vi "Channel Info by Index.vi"(8 "error in (no error)":errorcluster, 10 "Index":i32, 11 "GroupAbstract in":refnum<class "Group.lvclass">) -> (0 "error out":errorcluster, 2 "Channel Info":T1, 3 "GroupAbstract out":refnum<class "Group.lvclass">)   [LabVIEW 2020, in "Vecto.lvlib" / "Group.lvclass"]
uses:
  Group.lvclass
  Channel Info.ctl
  Group.lvclass/Group.ctl
  VectoConfig/VectoConfig.lvlib
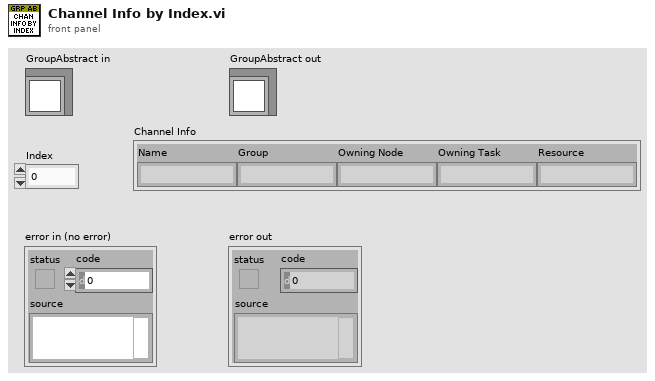
[diagram p1: front panel]
types:
  T1 = typedef "VectoConfig.lvlib/Channel Info.ctl" = cluster{"Name":string, "Group":string, "Owning Node":string, "Owning Task":string, "Resource":string}
  T2 = typedef "Vecto.lvlib/GroupAbstract.lvclass/Ref.ctl" = cluster{"Channel Index Map":map{string, i32}, "Channel Info":T3[]}
  T3 = typedef "Vecto.lvlib/Channel Info.ctl" = cluster{"Name":string, "Group":string, "Owning Node":string, "Owning Task":string, "Resource":string}
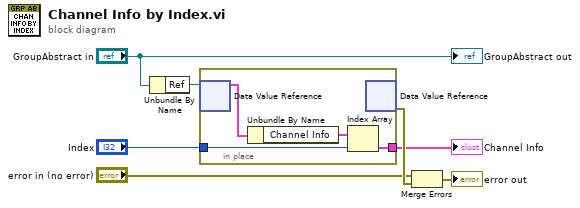
[diagram p0: block diagram]
diagram:
  n1 = Unbundle By Name("GroupAbstract in") -> ("Ref"=w6:refnum<data-value>)
  n2 = in-place {
    in-place-border: "Index" -> [w9]
    in-place-border: [w8] -> w4
    n3 = in-place-dvr #1(w6) -> (w11:T2)  [unwired: 1 out]
    n4 = Unbundle By Name(w11) -> ("Channel Info"=w10:T3[])
    n5 = Index Array(array=w10, index=w9) -> (element=w8:T3)
    n6 = in-place-dvr #1() -> (w7:errorcluster)  [unwired: 1 in, 1 out]
  }
  "Channel Info" <- w4
  n7 = Merge Errors("error in (no error)", w7) -> (→"error out":errorcluster)
  "GroupAbstract out" <- "GroupAbstract in"
